vi "PID_Wrapper.vi"(7 "output range":cluster{"output high":dbl, "output low":dbl}={"output high"=100.0, "output low"=-100.0} {"output low" format="%.2f"; "output high" format="%.2f"}, 9 "PID gains":T1={"proportional gain (Kc)"=1.0, "integral time (Ti, min)"=0.01, "derivative time (Td, min)"=0.0} {"derivative time (Td, min)" format="%.3f"; "integral time (Ti, min)" format="%.3f"; "proportional gain (Kc)" format="%.3f"}, 10 "process variable":dbl format="%.2f", 11 "setpoint":dbl format="%.2f") -> (3 "output":dbl format="%.2f")   [LabVIEW 2012]
uses:
  <vilib>/addons/control/pid/pid.llb/PID (DBL).vi
  <vilib>/addons/control/pid/NI_PID_pid.lvlib
panel:
  out "Time Difference":dbl
  in  "Reset":bool
  in  "Loop Iteration":i32
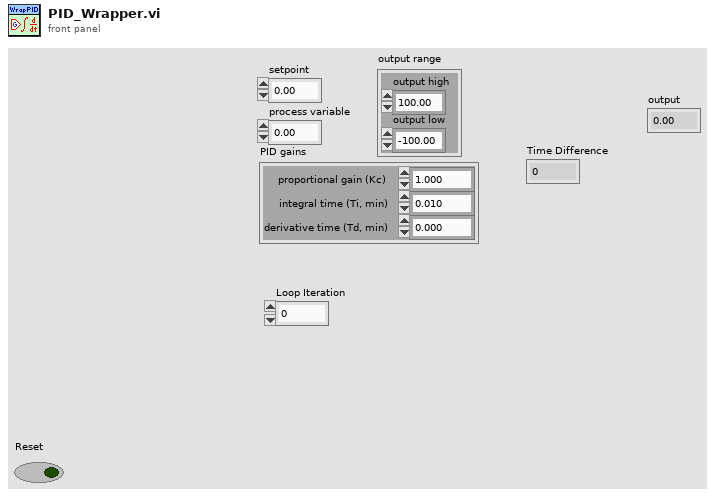
[diagram p1: front panel]
types:
  T1 = cluster{"proportional gain (Kc)":dbl, "integral time (Ti, min)":dbl, "derivative time (Td, min)":dbl}
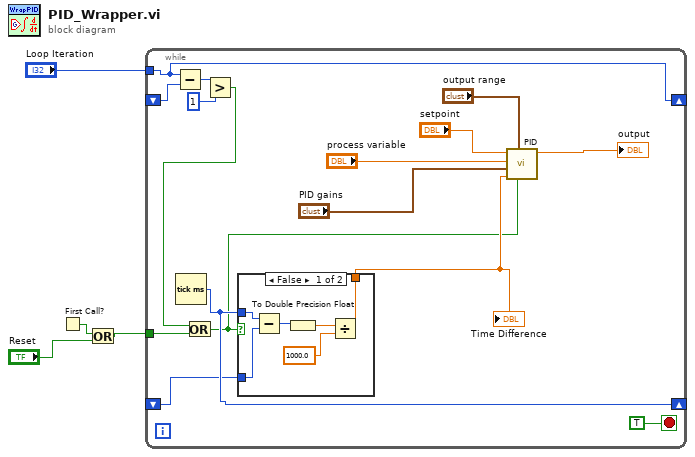
[diagram p0: block diagram]
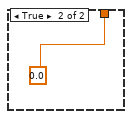
[diagram p2: hidden frame]
diagram:
  n1 = First Call?() -> (First Call?: T/F=w3:bool)
  n2 = Or(x=w3, y="Reset") -> (x .or. y?=w1:bool)
  n3 = while {
    shift-right: [w12] -> _
    shift-left: _ -> [w11]
    tunnel: "Loop Iteration" -> [w12]
    shift-right: [w10] -> _
    shift-left: _ -> [w9]
    tunnel: w1 -> [w8]
    stop <- TRUE stop-if-true
    n4 = Subtract(x=w12, y=w11) -> (x-y=w13:i32)
    n5 = Tick Count (ms)() -> (millisecond timer value=w10:u32)
    n6 = Greater?(x=w13, y=1) -> (0:w7:bool)
    n7 = Or(x=w7, y=w8) -> (x .or. y?=w5:bool)
    n8 = case shown="False" w5 {
      tunnel: w9 -> [w25 _]
      tunnel: w10 -> [w26 _]
      tunnel: [w23 0.0] -> w6
      frame False {
        n9 = Subtract(x=w26, y=w25) -> (x-y=w24:u32)
        n10 = To Double Precision Float(number=w24) -> (double precision float=w22:dbl)
        n11 = Divide(x=w22, y=1000.0) -> (x/y=w23:dbl)
      }
      frame True {
      }
    }
    "Time Difference" <- w6
    n12 = call-poly <vilib>:"PID.vi"("reinitialize? (F)"=w5, "output range"="output range", "dt (s)"=w6, "PID gains"="PID gains", "process variable"="process variable", "setpoint"="setpoint") -> ("output"=→"output":dbl)  [unwired: 4 in, 1 out]
  }
